vi "in_bounds.vi"(1 "Point":cluster{"X":i32, "Y":i32}, 2 "Ctl Refnum":refnum<vi>) -> (0 "In bounds":bool)   [LabVIEW 2017]
panel:
  # "This VI takes a Dimension (width and height ) and a point (x and y) and tells whether or not the point is in the box."
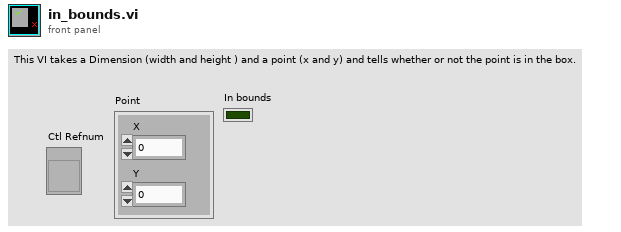
[diagram p1: front panel]
types:
  T1 = typedef "LVBoundsTypeDef.ctl" = cluster{"Width":u32, "Height":u32}
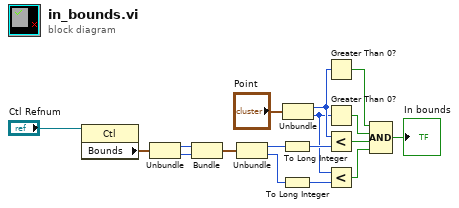
[diagram p0: block diagram]
diagram:
  n1 = property class="Ctl"(reference="Ctl Refnum") -> ("Bounds"=w5:T1)  [unwired: 1 in, 2 out]
  n2 = Unbundle(w5) -> ("Width"=w4:u32, "Height"=w3:u32)
  n3 = Bundle("Width"=w4, "Height"=w3) -> (w1:cluster{"Width":u32, "Height":u32})  [unwired: 1 in]
  n4 = Unbundle(w1) -> ("Width"=w7:u32, "Height"=w6:u32)
  n5 = To Long Integer(number=w7) -> (32bit integer=w16:i32)
  n6 = To Long Integer(number=w6) -> (32bit integer=w15:i32)
  n7 = Unbundle("Point") -> ("X"=w9:i32, "Y"=w8:i32)
  n8 = Greater Than 0?(x=w9) -> (x > 0?=w14:bool)
  n9 = Greater Than 0?(x=w8) -> (x > 0?=w13:bool)
  n10 = Less?(x=w9, y=w16) -> (x < y?=w10:bool)
  n11 = Less?(x=w8, y=w15) -> (x < y?=w12:bool)
  n12 = Compound Arithmetic op=AND(w14, w13, w10, w12) -> (→"In bounds":bool)
